vi "项操作.vi"(8 "error in (no error)":errorcluster caption="错误输入（无错误）", 9 "Cell Position":T1, 10 "MCListbox引用句柄":refnum<vi>, 11 "Delete 输入":refnum<class "Delete.lvclass">) -> (0 "error out":errorcluster caption="错误输出", 3 "Delete 输出":refnum<class "Delete.lvclass">)   [LabVIEW 2016, in "Delete.lvclass"]
uses:
  Delete.lvclass
  <vilib>/Utility/miscctls.llb/LVRowAndColumnTypeDef.ctl
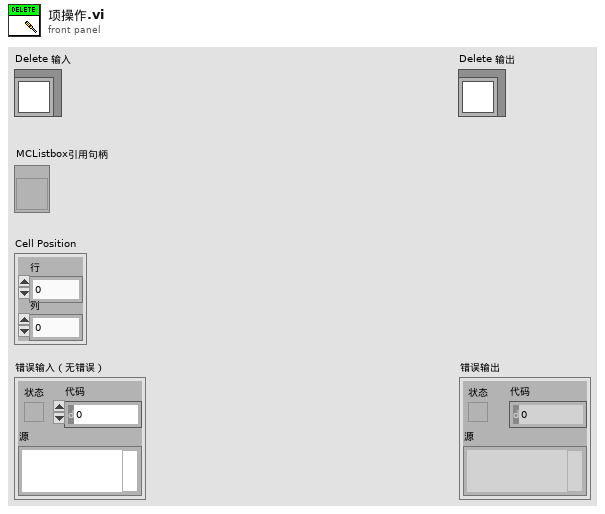
[diagram p1: front panel]
types:
  T1 = typedef "LVRowAndColumnTypeDef.ctl" = cluster{"Row":i32, "Column":i32}
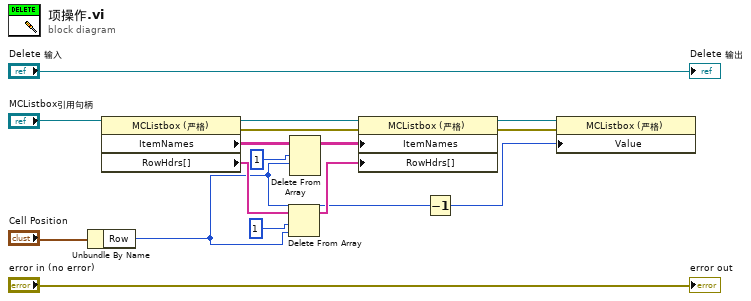
[diagram p0: block diagram]
diagram:
  n1 = Unbundle By Name("Cell Position") -> ("Row"=w1:i32)
  n2 = property class="MCListbox (严格)"(reference="MCListbox引用句柄") -> (reference out=w13:refnum<vi>, error out=w12:errorcluster, "ItemNames"=w11:string[][], "RowHdrs[]"=w4:string[])  [unwired: 1 in]
  n3 = Delete From Array(array=w4, length=1 ("长度"), index=w1) -> (array with subset deleted=w3:string[])  [unwired: 1 out]
  n4 = Delete From Array(array=w11, length=1 ("长度"), index (row)=w1) -> (array with subset deleted=w9:string[][])  [unwired: 1 in, 1 out]
  n5 = property class="MCListbox (严格)"(reference=w13, error in=w12, "ItemNames"=w9, "RowHdrs[]"=w3) -> (reference out=w8:refnum<vi>, error out=w7:errorcluster)
  n6 = Decrement(x=w1) -> (x-1=w6:i32)
  n7 = property class="MCListbox (严格)"(reference=w8, error in=w7, "Value"=w6) -> ()  [unwired: 2 out]
  "error out" <- "error in (no error)"
  "Delete 输出" <- "Delete 输入"
